vi "spi_16b_master.vi"(7 "Falling Edge?":bool=TRUE, 8 "SIG Port":refnum<k21>="Connector0/DIO0", 9 "CLK Port":refnum<k21>="Connector0/DIO1", 11 "SPI data  (MSB First)":u16) -> ()   [LabVIEW 2010, in "kevLib2010.lvlib"]
uses:
  kevLib2010.lvlib
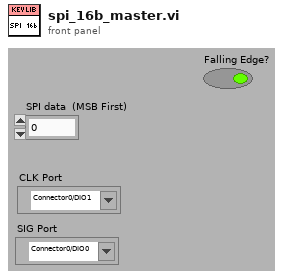
[diagram p1: front panel]
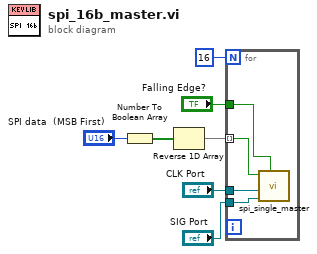
[diagram p0: block diagram]
diagram:
  n1 = Number To Boolean Array(number="SPI data  (MSB First)") -> (Boolean array=w6:bool[])
  n2 = Reverse 1D Array(array=w6) -> (reversed array=w5:bool[])
  n3 = for {
    N: 16 -> [_]
    tunnel: w5 -> [w11] mode=indexing
    tunnel: "CLK Port" -> [w10]
    tunnel: "SIG Port" -> [w9]
    tunnel: "Falling Edge?" -> [w8]
    n4 = call "spi_single_master.vi"("Falling Edge?"=w8, "SIG Port"=w9, "CLK Port"=w10, "Signal"=w11) -> ()  [unwired: 6 in, 2 out]
  }
